vi "RSZVB Set Power Meter Frequency Conversion.vi"(4 "Numerator (1)":i32=1, 5 "Sweep Type (0: Sweep)":i32(ring) items=["Sweep", "CW/Fixed"], 6 "Offset (0.0)":dbl format="%^.3e", 7 "Denominator (1)":i32=1, 8 "error in (no error)":errorcluster {"code" format="%.0x"}, 9 "Power Meter Number (1)":i32=1, 10 "Channel (1)":i32=1, 11 "VISA session":refnum<visa-resource-name>) -> (0 "error out":errorcluster {"code" format="%.0x"}, 3 "dup VISA session":refnum<visa-resource-name>)   [LabVIEW 2011]
doc: "This VI defines the receiver frequency for frequency-converting measurements. The receiver frequency is either a range (for frequency sweeps) or a CW frequency (for power, time and CW Mode sweeps). The receiver frequency is valid for all ports. \n\nNote(s):\n\n(1) This VI is available only on R&S ZVA instrument.\n\nRemote-control command(s):\n[SENSe<Ch>:]FREQuency:CONVersion:ARBitrary:PMETer<Mtr> <numerator>, <denominator>, <offset>, CW | FIXed | SWEep"
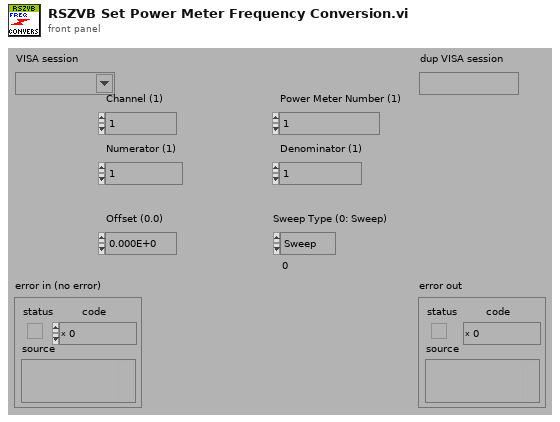
[diagram p1: front panel]
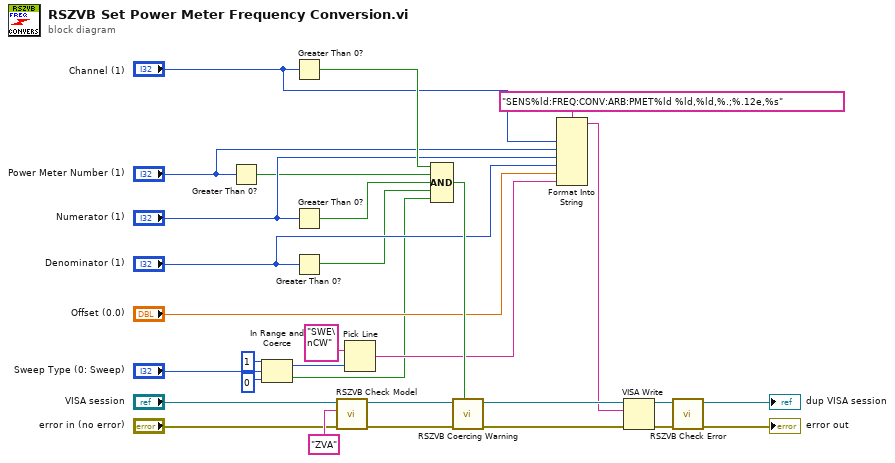
[diagram p0: block diagram]
diagram:
  n1 = Greater Than 0?(x="Power Meter Number (1)") -> (x > 0?=w6:bool)
  n2 = In Range and Coerce(upper limit=1 ("lower limit"), x="Sweep Type (0: Sweep)", lower limit=0) -> (coerced(x)=w22:i32, In Range?=w1:bool)
  n3 = Greater Than 0?(x="Channel (1)") -> (x > 0?=w30:bool)
  n4 = Greater Than 0?(x="Numerator (1)") -> (x > 0?=w7:bool)
  n5 = Greater Than 0?(x="Denominator (1)") -> (x > 0?=w8:bool)
  n6 = call "RSZVB Check Model.vi"("error in (no error)"="error in (no error)", "Model"="ZVA" ("Options"), "VISA session"="VISA session") -> ("error out"=w19:errorcluster, "dup VISA session"=w18:refnum<visa-resource-name>)  [unwired: 7 in]
  n7 = Pick Line(multi-line string="SWE\nCW", line index=w22) -> (output string=w15:string)  [unwired: 1 in]
  n8 = Compound Arithmetic op=AND(w30, w6, w7, w8, w1) -> (w29:bool)
  n9 = call "RSZVB Coercing Warning.vi"("In Range?"=w29, "error in (no error)"=w19, "VISA session"=w18) -> ("error out"=w21:errorcluster, "dup VISA session"=w26:refnum<visa-resource-name>)  [unwired: 7 in]
  n10 = Format Into String(format string="SENS%ld:FREQ:CONV:ARB:PMET%ld %ld,%ld,%.;%.12e,%s", "Channel (1)", "Power Meter Number (1)", "Numerator (1)", "Denominator (1)", "Offset (0.0)", w15) -> (resulting string=w16:string)  [unwired: 2 in, 1 out]
  n11 = VISA Write(VISA resource name=w26, write buffer=w16, error in (no error)=w21) -> (VISA resource name out=w28:refnum<visa-resource-name>, error out=w27:errorcluster)  [unwired: 1 out]
  n12 = call "RSZVB Check Error.vi"("error in (no error)"=w27, "VISA session"=w28) -> ("error out"=→"error out":errorcluster, "dup VISA session"=→"dup VISA session":refnum<visa-resource-name>)  [unwired: 8 in]
